vi "speedTransformation.vi"(0 "Game in":refnum<class "Game.lvclass">, 1 "V_norm_limit":dbl format="%#_13g", 2 "Vang_limit":dbl=4.0, 3 "PID Gains Angle":T1={"proportional gain (Kc)"=3.0, "integral time (Ti, min)"=0.0, "derivative time (Td, min)"=2.0}, 5 "Robot":refnum<class "Robot.lvclass">, 7 "DistToDestOrientation":dbl=1000.0 format="%#_13g", 9 "Dest":dbl[](array[numeric])=[4500.0, 3000.0] format="%#_13g", 11 "error in (no error)":errorcluster, 12 "V_sent":dbl=3.0 format="%#_13g", 14 "last_dest":bool=TRUE) -> (4 "Game out":refnum<class "Game.lvclass">, 6 "Robot out":refnum<class "Robot.lvclass">, 15 "error out":errorcluster)   [LabVIEW 2020, in "Game.lvclass"]
uses:
  Game.lvclass
  Robot_class/Robot.lvclass
  C:/RoboIME/SSL_AI/Object_class/Object.lvclass
  Object_class/Object.lvclass/Object.ctl
  Robot_class/Robot.lvclass/Robot.ctl
  <vilib>/Analysis/baseanly.llb/Unit Vector (DBL).vi
  <vilib>/Analysis/coordinate.llb/2D Cartesian Coordinate Rotation (Scalar).vi
  Object_class/Read x.vi
  Object_class/Read y.vi
  Robot_class/Read orientation.vi
  Robot_class/Write v_tang.vi
  Robot_class/Write v_norm.vi
  Robot_class/Write v_ang.vi
  <vilib>/Analysis/NI_AALPro.lvlib
  <vilib>/Analysis/NI_AALBase.lvlib
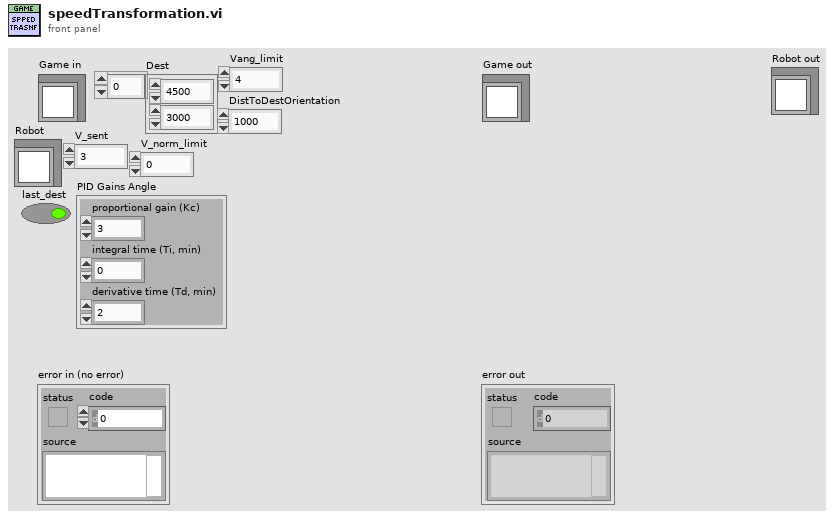
[diagram p1: front panel]
types:
  T1 = cluster{"proportional gain (Kc)":dbl, "integral time (Ti, min)":dbl, "derivative time (Td, min)":dbl}
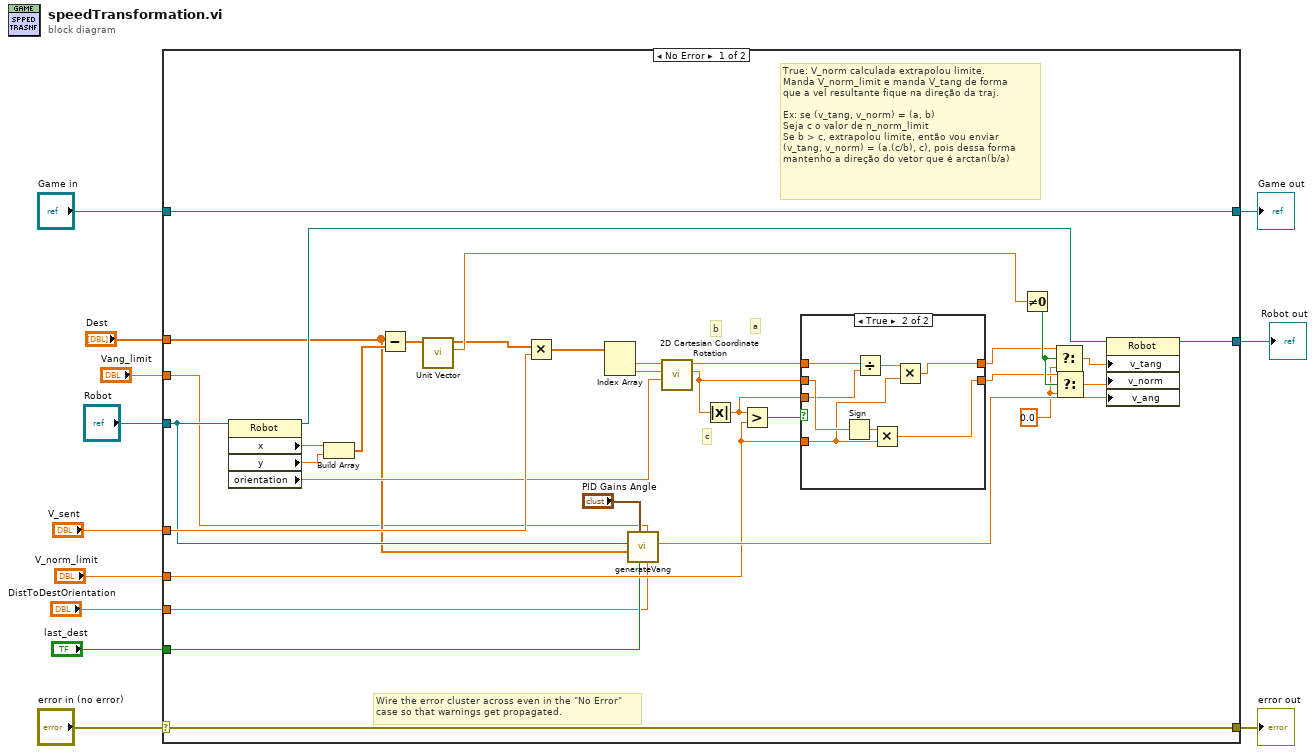
[diagram p0: block diagram]
diagram:
  n1 = case shown="No Error" "error in (no error)" {
    selector: "error in (no error)" -> [w44 w57]
    tunnel: [w44 w57] -> w11
    tunnel: [w45 w56] -> w9
    tunnel: "Game in" -> [w45 w56]
    tunnel: "Robot" -> [w31 _]
    tunnel: "Dest" -> [w25 _]
    tunnel: "V_sent" -> [w40 _]
    tunnel: [w35 _] -> w5
    tunnel: "V_norm_limit" -> [w27 _]
    tunnel: "last_dest" -> [w24 _]
    tunnel: "Vang_limit" -> [w14 _]
    tunnel: "DistToDestOrientation" -> [w13 _]
    frame No Error {
      w19 = 0.0
      # "c"
      # "a"
      # "b"
      # "True: V_norm calculada extrapolou limite.\nManda V_norm_limit e manda V_tang de forma\nque a vel resultante fique na direção da traj.\n\nEx: se (v_tang, v_norm) = (a, b)\nSeja c o valor de n_norm_limit\nSe b > c, extrapolou limite, então vou enviar \n(v_tang, v_norm) = (a.(c/b), c), pois dessa forma \nmantenho a direção do vetor que é arctan(b/a)"
      # "Wire the error cluster across even in the \"No Error\"\ncase so that warnings get propagated."
      n2 = property class="Robot"(reference=w31) -> (reference out=w36:refnum<class "Robot.lvclass">, "x"=w43:dbl, "y"=w42:dbl, "orientation"=w33:dbl)  [unwired: 1 in, 1 out]
      n3 = Build Array(w43, w42) -> (w41:dbl[])
      n4 = Subtract(x=w25, y=w41) -> (x-y=w15:dbl[])
      n5 = call-poly <vilib>:"Unit Vector.vi"("Input Vector"=w15) -> ("norm"=w17:dbl, "Unit Vector"=w16:dbl[])  [unwired: 8 in, 1 out]
      n6 = Multiply(x=w16, y=w40) -> (x*y=w39:dbl[])
      n7 = Index Array(array=w39) -> (element #1=w38:dbl, element #2=w37:dbl)  [unwired: 2 in]
      n8 = call "generateVang.vi"("DistToDestOrientation"=w13, "Vang_limit"=w14, "last_dest"=w24, "PID Gains Angle"="PID Gains Angle", "Dest"=w25, "Robot"=w31) -> ("Vang"=w32:dbl)  [unwired: 3 in, 2 out]
      n9 = call-poly <vilib>:"2D Cartesian Coordinate Rotation.vi"("theta"=w33, "y"=w37, "x"=w38) -> ("y out"=w28:dbl, "x out"=w29:dbl)  [unwired: 6 in, 1 out]
      n10 = Absolute Value(x=w28) -> (abs(x)=w26:dbl)
      n11 = Greater?(x=w26, y=w27) -> (0:w30:bool)
      n12 = case shown="True" w30 {
        tunnel: [w47 w48] -> w21
        tunnel: w29 -> [w47 w52]
        tunnel: [w46 w53] -> w20
        tunnel: w28 -> [w46 w55]
        tunnel: w27 -> [_ w49]
        tunnel: w26 -> [_ w51]
        frame False {
        }
        frame True {
          n13 = Sign(1:w55) -> (0:w54:dbl)
          n14 = Divide(x=w52, y=w51) -> (x/y=w50:dbl)
          n15 = Multiply(x=w54, y=w49) -> (x*y=w53:dbl)
          n16 = Multiply(x=w50, y=w49) -> (x*y=w48:dbl)
        }
      }
      n17 = Not Equal To 0?(x=w17) -> (x != 0?=w22:bool)
      n18 = Select(t=w21, s=w22, f=w19) -> (s? t:f=w23:dbl)
      n19 = Select(t=w20, s=w22, f=w19) -> (s? t:f=w18:dbl)
      n20 = property class="Robot"(reference=w36, "v_tang"=w23, "v_norm"=w18, "v_ang"=w32) -> (reference out=w35:refnum<class "Robot.lvclass">)  [unwired: 1 in, 1 out]
    }
    frame Error {
    }
  }
  "error out" <- w11
  "Game out" <- w9
  "Robot out" <- w5
